vi "Read Measurement.vi"(8 "error in":errorcluster, 10 "call id in":T1, 11 "gRPCid in":T1) -> (0 "error out":errorcluster, 1 "measurement results":T2, 2 "call id out":T1, 3 "gRPCid out":T1, 5 "measure success?":bool)   [LabVIEW 2021, in "MeasurementServerTests.lvlib" / "Measurement Service Tests.lvlib" / "Continuous Counting Client.lvlib"]
doc: "Read and unpack the measurement results, until the measurement fails."
uses:
  Continuous Counting Client.lvlib
  <vilib>/gRPC/LabVIEW gRPC Library/Shared/grpcId.ctl
  controls/Measurement Results.ctl
  34829905-00c5-4e32-9a4f-e87a22ec28de.vi
  <vilib>/gRPC/LabVIEW gRPC Library/Server API/Translate Protobuf Error.vi
  <vilib>/AdvancedString/1D String Array to Delimited String.vi
  <vilib>/gRPC/LabVIEW gRPC Library/Server API/Server/Get Server DLL Path.vi
  gRPC/Generated APIs/ni/measurementlink/measurement/v2/Measurement Service Client V2/Measurement Service Client V2.lvlib
  <vilib>/gRPC/LabVIEW gRPC Library/grpc-lvsupport-release.lvlib
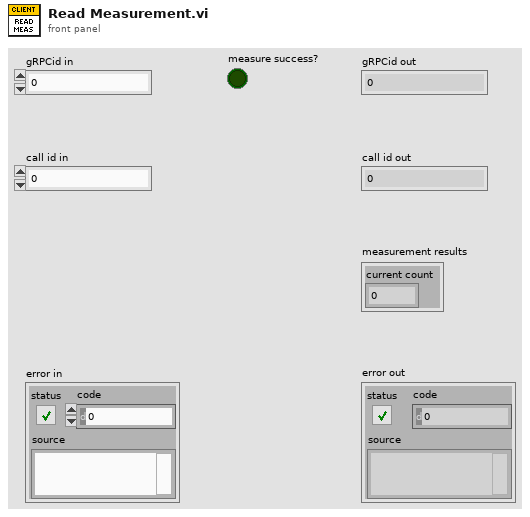
[diagram p1: front panel]
types:
  T1 = typedef "grpc-lvsupport-release.lvlib/grpcId.ctl" = u64
  T2 = typedef "MeasurementServerTests.lvlib/Measurement Service Tests.lvlib/Continuous Counting Client.lvlib/Measurement Results.ctl" = cluster{"current count":i64}
  T3 = typedef "Measurement Service Client V2.lvlib/ni_measurementlink_measurement_v2_MeasureResponse.ctl" = cluster{"outputs":T4}
  T4 = typedef "Measurement Service Client V2.lvlib/google_protobuf_Any.ctl" = cluster{"type_url":string, "value":u8[]}
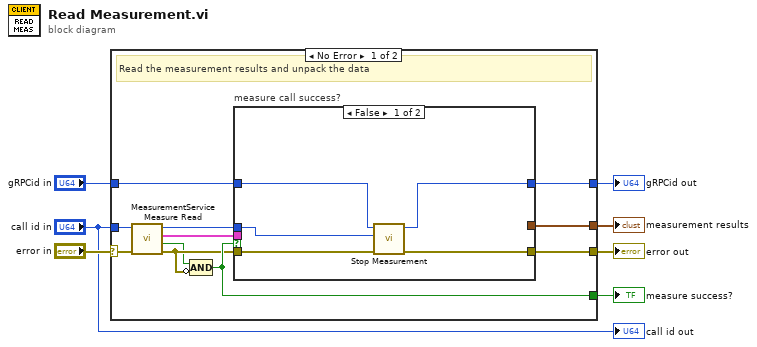
[diagram p0: block diagram]
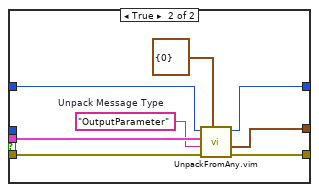
[diagram p2: hidden frame]
diagram:
  n1 = case shown="No Error" "error in" {
    selector: "error in" -> [w13 w32]
    tunnel: "gRPCid in" -> [w18 w33]
    tunnel: "call id in" -> [w12 _]
    tunnel: [w17 _] -> w6
    tunnel: [w16 w33] -> w5
    tunnel: [w15 w32] -> w4
    tunnel: [w14 _] -> w3
    frame No Error {
      # "Read the measurement results and unpack the data"
      n2 = call "MeasurementService Measure Read.vi"("error in"=w13, "Call ID in"=w12) -> ("error out"=w9:errorcluster, "Success"=w8:bool, "Response Data"=w11:T3, "Call ID"=w10:T1)  [unwired: 6 in]
      n3 = Compound Arithmetic op=AND(w8, invert w9) -> (w14:bool)
      n4 = case "measure call success?" shown="False" w14 {
        tunnel: w11 -> [_ w31]
        tunnel: [w22 w30] -> w15
        tunnel: w9 -> [w23 w29]
        tunnel: [w19 w27] -> w16
        tunnel: [_ w25] -> w17
        tunnel: w18 -> [w20 w24]
        tunnel: w10 -> [w21 _]
        frame False {
          n5 = call "Stop Measurement.vi"("error in"=w23, "call id"=w21, "gRPCid in"=w20) -> ("error out"=w22:errorcluster, "gRPCid out"=w19:T1)  [unwired: 7 in]
        }
        frame True {
          w26 = "OutputParameter"  # Unpack Message Type
          n6 = call "UnpackFromAny.vim"("Data Type"=T2 {"current count"=0} ("measurement results"), "error in"=w29, "Message Type"=w26, "Any"=w31, "gRPCid in"=w24) -> ("error out"=w30:errorcluster, "Unpacked Value"=w25:T2, "gRPCid out"=w27:u64)  [unwired: 4 in]
        }
      }
    }
    frame Error {
      # "Pass"
    }
  }
  "measurement results" <- w6
  "gRPCid out" <- w5
  "error out" <- w4
  "measure success?" <- w3
  "call id out" <- "call id in"
